vi "LVObject to JSON - Array of Object - Returns JSON String.vi"() -> ()   [LabVIEW 2017, in "Generic Object Serializer Tests.lvlib"]
uses:
  Generic Object Serializer Tests.lvlib
  Generic Object Serializer/Generic Object Serializer.lvclass
  <vilib>/addons/_JKI Toolkits/Caraya/classes/Assert/Assert Equal Value_Variant.vi
  <vilib>/addons/_JKI Toolkits/Caraya/classes/Test/Test.lvclass
  <vilib>/addons/_JKI Toolkits/Caraya/classes/Assert/Assert.lvclass
  Country/Country.lvclass
panel:
  out "error out":errorcluster
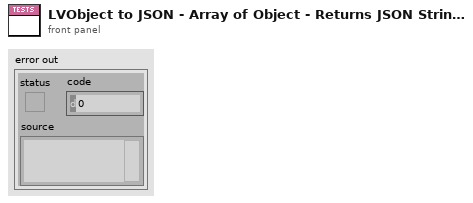
[diagram p1: front panel]
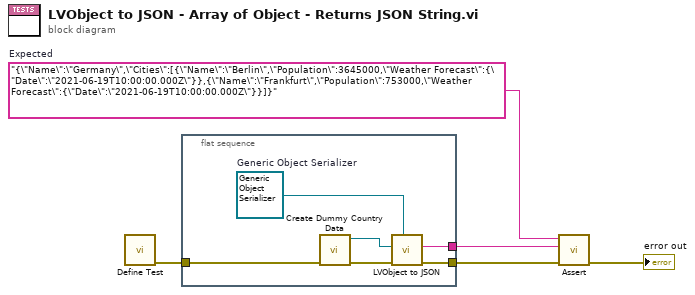
[diagram p0: block diagram]
diagram:
  w1 = "{\"Name\":\"Germany\",\"Cities\":[{\"Name\":\"Berlin\",\"Population\":3645000,\"Weather Forecast\":{\"Date\":\"2021-06-19T10:00:00.000Z\"}},{\"Name\":\"Frankfurt\",\"Population\":753000,\"Weather Forecast\":{\"Date\":\"2021-06-19T10:00:00.000Z\"}}]}"  # Expected
  n1 = call <vilib>:"Define Test.vi"() -> ("error out"=w4:errorcluster)  [unwired: 11 in]
  n2 = flat-sequence {
    tunnel: w4 -> [w7]
    tunnel: [w9] -> w3
    tunnel: [w10] -> w2
    frame #0 {
      w11 = refnum<class "Generic Object Serializer.lvclass"> refnum  # Generic Object Serializer
      n3 = call "Create Dummy Country Data.vi"("error in (no error)"=w7) -> ("error out"=w8:errorcluster, "Country"=w6:refnum<class "Country.lvclass">)  [unwired: 9 in]
      n4 = call-dynamic "LVObject to JSON.vi"("LVClass Serializer"=w11, "error in (no error)"=w8, "Object"=w6) -> ("error out"=w9:errorcluster, "<JSON>Object"=w10:string)  [unwired: 7 in]
    }
  }
  n5 = call-poly <vilib>:"Assert.vi"("error in (no error)"=w3, "Y"=w2, "X"=w1) -> ("error out"=→"error out":errorcluster)  [unwired: 8 in]
